vi "stop_sbig.vi"(2 "path":path) -> (0 "error out":errorcluster)   [LabVIEW 2018]
panel:
  out "appended path":path
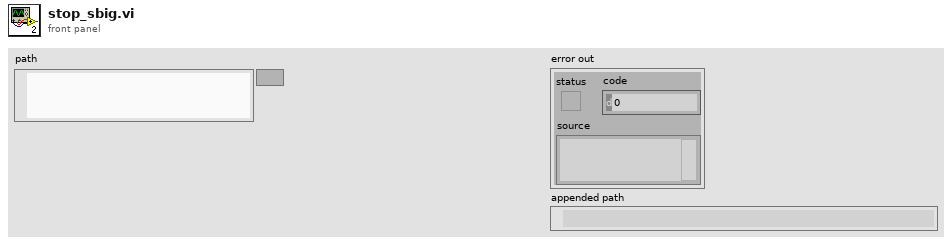
[diagram p1: front panel]
types:
  T1 = enum16{"open", "replace", "create", "open or create", "replace or create", "replace or create with confirmation"}
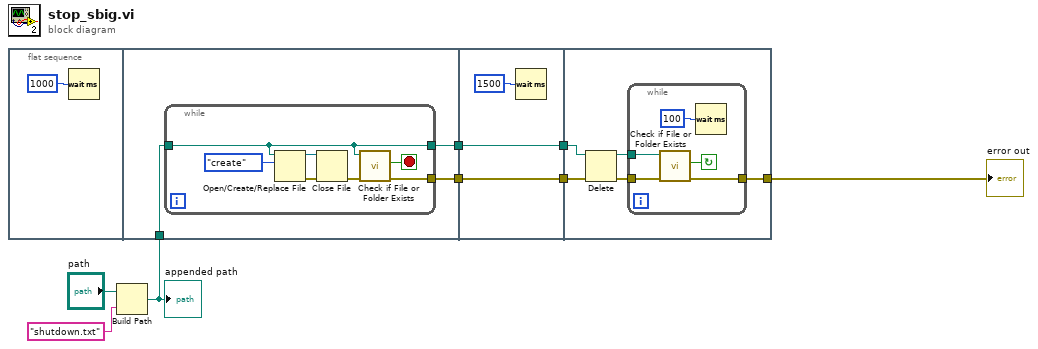
[diagram p0: block diagram]
diagram:
  n1 = flat-sequence {
    tunnel: w6 -> [w12]
    tunnel: [w11] -> w5
    tunnel: [w10] -> w4
    tunnel: [w21] -> w2
    tunnel: w5 -> [w21]
    tunnel: [w20] -> w1
    tunnel: w4 -> [w20]
    tunnel: w2 -> [w26]
    tunnel: w1 -> [w24]
    tunnel: [w27] -> w3
    frame #0 {
      n2 = Wait (ms)(milliseconds to wait=u32 1000) -> ()  [unwired: 1 out]
    }
    frame #1 {
      n3 = while {
        tunnel: w12 -> [w16]
        tunnel: [w16] -> w11
        tunnel: [w18] -> w10
        stop <- w19 stop-if-true
        n4 = Open/Create/Replace File(file path (use dialog)=w16, operation (0:open)=T1."create") -> (refnum out=w17:refnum<file>, error out=w15:errorcluster)  [unwired: 4 in, 1 out]
        n5 = Close File(refnum=w17, error in=w15) -> (error out=w14:errorcluster)  [unwired: 1 out]
        n6 = call <vilib>:"Check if File or Folder Exists.vi"("error in (no error)"=w14, "path"=w16) -> ("error out"=w18:errorcluster, "file or folder exists?"=w19:bool)  [unwired: 7 in, 1 out]
      }
    }
    frame #2 {
      n7 = Wait (ms)(milliseconds to wait=u32 1500) -> ()  [unwired: 1 out]
    }
    frame #3 {
      n8 = Delete(path (use dialog)=w26, error in=w24) -> (deleted path=w25:path, error out=w23:errorcluster)  [unwired: 3 in, 1 out]
      n9 = while {
        tunnel: w25 -> [w30]
        tunnel: w23 -> [w29]
        tunnel: [w28] -> w27
        stop <- w32 continue-if-true
        n10 = call <vilib>:"Check if File or Folder Exists.vi"("error in (no error)"=w29, "path"=w30) -> ("error out"=w28:errorcluster, "file or folder exists?"=w32:bool)  [unwired: 7 in, 1 out]
        n11 = Wait (ms)(milliseconds to wait=u32 100) -> ()  [unwired: 1 out]
      }
    }
  }
  n12 = Build Path(base path="path", name or relative path="shutdown.txt") -> (appended path=w6:path)
  "appended path" <- w6
  "error out" <- w3
